vi "HDI Accuracy.vi"() -> ()   [LabVIEW 2011]
uses:
  Shared Components/Gantry Class/Type Definitions/Virtual Modes.ctl
  Shared Components/Gantry Class/Type Definitions/Init_Modes.ctl
  Shared Components/Gantry Class/Gantry Class.lvclass
  Shared Components/Config Manager Class/Type Definitions/Camera Enum.ctl
  Shared Components/Vec3d Class/Vec3d Class.lvclass
panel:
  out "Point being recorded":string="\\P"
  in  "Results Folder":path=path "C:/Users/Admin/Gantry Purdue/pixel-gantry-control/Results"
  out "Iteration Number":i32
  in  "Virtual Mode":T1=enum."Virtual"
  in  "stop":bool
  out "Image":T2(plugin-control)
  out "error out":errorcluster
  in  "Config Folder":path=path "C:/Users/Admin/Gantry Purdue/pixel-gantry-control/Config"
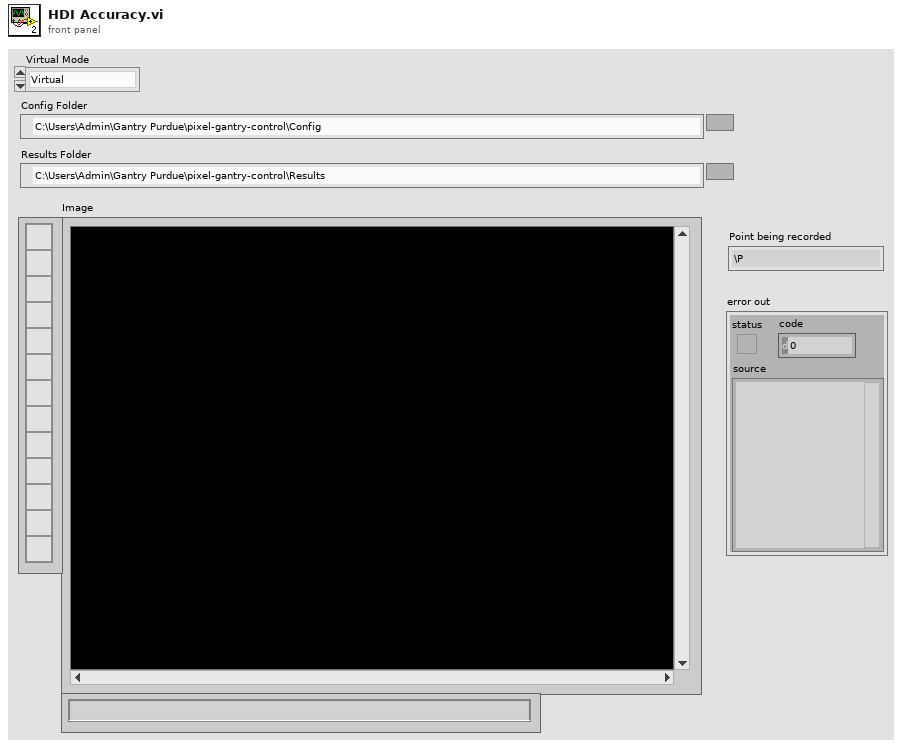
[diagram p1: front panel]
types:
  T1 = typedef "Virtual Modes.ctl" = enum16{"Nonvirtual", "Pseudovirtual", "Virtual"}
  T2 = typedef "IMAQ Image.ctl" = refnum<image>
  T3 = typedef "Init_Modes.ctl" = enum16{"Full", "Robot Only", "Dispenser Only", "Cameras Only", "Robot and Cameras", "Robot and Cameras and Dispenser", "Manifold Only"}
  T4 = typedef "Camera Enum.ctl" = enum16{"GANTRY HEAD", "NEEDLE CALIBRATION X", "NEEDLE CALIBRATION Y", "STAND CAMERA", "SIMRAN WEBCAM"}
  T5 = typedef "Physical Image.ctl" = cluster{"Image Position":refnum<class "Vec3d Class.lvclass">, "Image Reference":T2, "Field of View":cluster{"x(mm)":dbl, "y(mm)":dbl}}
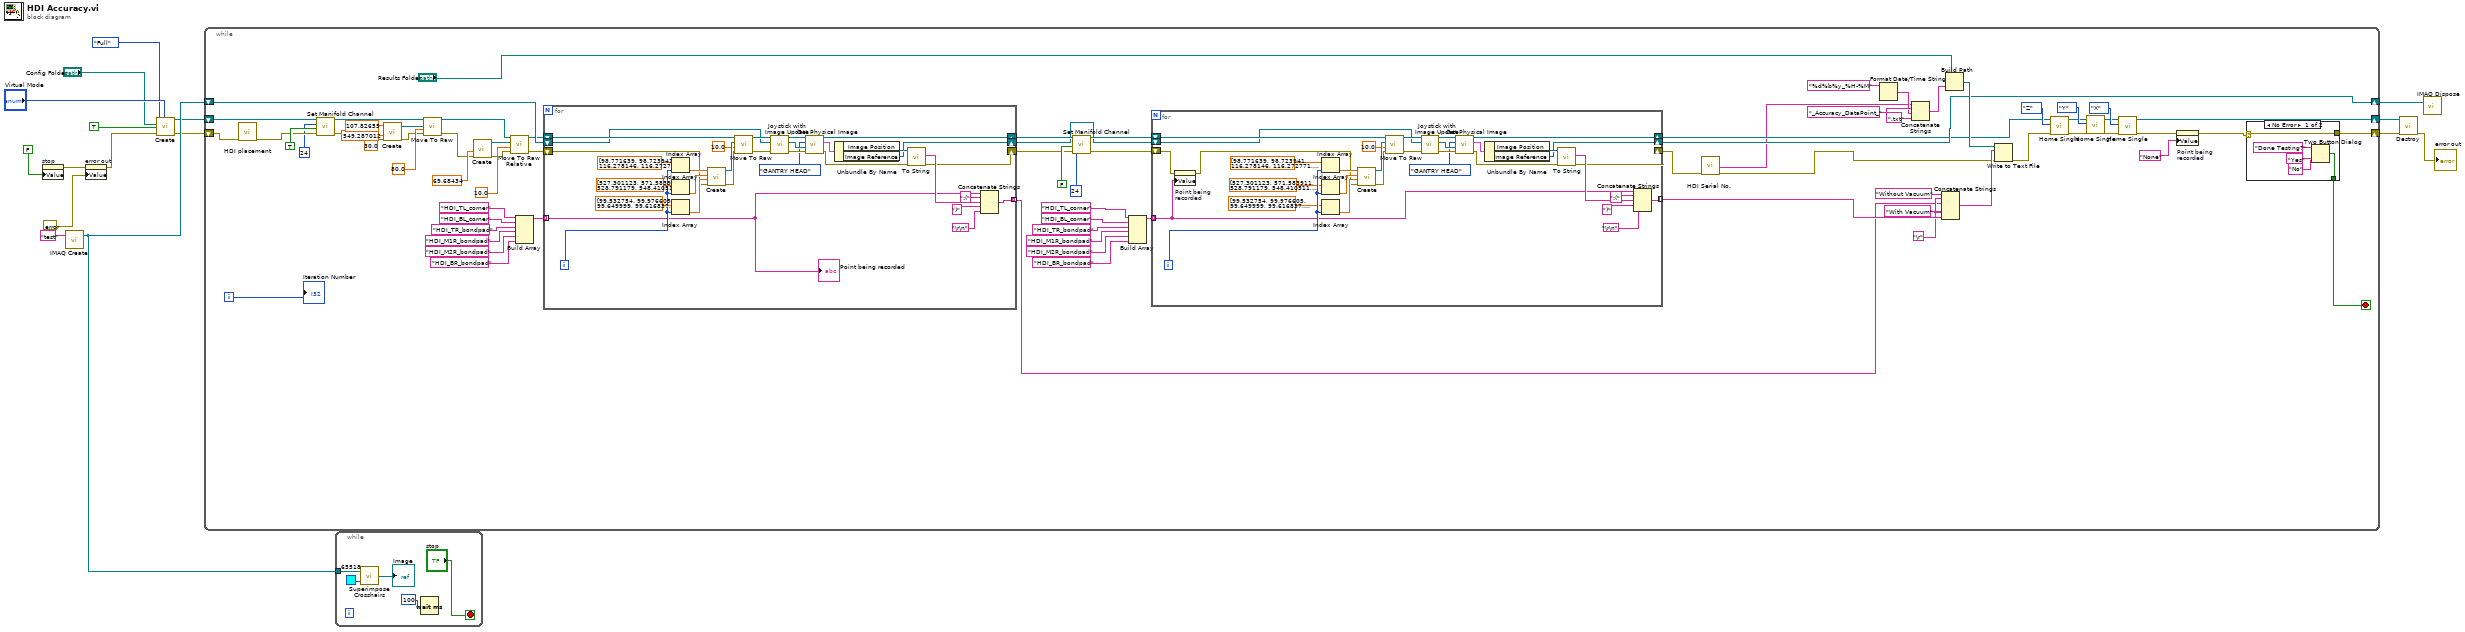
[diagram p0: block diagram]
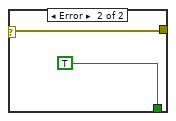
[diagram p2: hidden frame]
diagram:
  n1 = property on="stop" class="Bool (strict)"("Value"=FALSE) -> (error out=w14:errorcluster)  [unwired: 2 in, 1 out]
  n2 = call "IMAQ Create"("Image Name"="test") -> ("New Image"=w11:T2)  [unwired: 4 in, 1 out]
  n3 = property on="error out" class="Clust (strict)"(error in=w14, "Value"=errorcluster {"status"=FALSE, "code"=0, "source"=""} ("error in (no error)")) -> (error out=w9:errorcluster)  [unwired: 1 in, 1 out]
  n4 = call "Create.vi"("Virtual Mode"="Virtual Mode", "error in"=w9, "HOME?"=TRUE, "Config Folder"="Config Folder", "Init Mode"=Init_Modes."Full") -> ("error out"=w6:errorcluster, "Gantry out"=w5:refnum<class "Gantry Class.lvclass">)  [unwired: 5 in]
  n5 = while {
    shift-right: [w34] -> w3
    shift-left: w11 -> [w49]
    shift-right: [w71] -> w2
    shift-left: w5 -> [w76]
    shift-right: [w70] -> w1
    shift-left: w6 -> [w57]
    i -> [w78]
    stop <- w79 stop-if-true
    w37 = "\r"
    n6 = call "HDI placement"("error in (no error)"=w57) -> ("error out"=w74:errorcluster)  [unwired: 17 in, 1 out]
    n7 = call-dynamic "Set Manifold Channel.vi"("error in"=w74, "On/Off"=TRUE, "Manifold Channel"=24, "Gantry in"=w76) -> ("error out"=w73:errorcluster, "Gantry out"=w75:refnum<class "Gantry Class.lvclass">)  [unwired: 6 in]
    n8 = call "Create.vi"("error in"=w73, "Z"=30.0, "Y"=549.287012, "X"=107.82655) -> ("error out"=w89:errorcluster, "Vec3d Class out"=w91:refnum<class "Vec3d Class.lvclass">)  [unwired: 6 in]
    n9 = call-dynamic "Move To Raw.vi"("error in"=w89, "Speed"=80.0, "Destination"=w91, "Gantry in"=w75) -> ("error out"=w47:errorcluster, "Gantry out"=w50:refnum<class "Gantry Class.lvclass">)  [unwired: 6 in]
    n10 = call "Create.vi"("error in"=w47, "Z"=69.68434) -> ("error out"=w58:errorcluster, "Vec3d Class out"=w61:refnum<class "Vec3d Class.lvclass">)  [unwired: 8 in]
    n11 = call-dynamic "Move To Raw Relative.vi"("error in"=w58, "Speed(mm/s)"=10.0, "Delta"=w61, "Gantry in"=w50) -> ("error out"=w48:errorcluster, "Gantry out"=w27:refnum<class "Gantry Class.lvclass">)  [unwired: 6 in]
    n12 = Build Array("HDI_TL_corner" ("string"), "HDI_BL_corner" ("string"), "HDI_TR_bondpad" ("string"), "HDI_M1R_bondpad" ("string"), "HDI_M2R_bondpad" ("string"), "HDI_BR_bondpad" ("string")) -> (w63:string[])
    n13 = for {
      tunnel: [w155] -> w35 mode=indexing
      shift-right: [w156] -> w24
      shift-left: w48 -> [w133]
      shift-right: [w154] -> w22
      shift-left: w27 -> [w149]
      shift-right: [w150] -> w17
      shift-left: w49 -> [w138]
      tunnel: w63 -> [w132] mode=indexing
      i -> [w134]
      n14 = Index Array(array=dbl[] [98.771639, 98.723941, 116.278146, 116.272771, 116.262135, 116.231002, 0.0, 0.0], index=w134) -> (element=w146:dbl)
      n15 = Index Array(array=dbl[] [527.301123, 571.583911, 528.791179, 548.410511, 550.612629, 570.266275, 0.0, 0.0], index=w134) -> (element=w145:dbl)
      n16 = Index Array(array=dbl[] [99.532754, 99.976605, 99.649999, 99.616837, 99.684329, 99.659099, 0.0, 0.0], index=w134) -> (element=w136:dbl)
      n17 = call "Create.vi"("error in"=w133, "Z"=w136, "Y"=w145, "X"=w146) -> ("error out"=w143:errorcluster, "Vec3d Class out"=w144:refnum<class "Vec3d Class.lvclass">)  [unwired: 6 in]
      n18 = call-dynamic "Move To Raw.vi"("error in"=w143, "Speed"=10.0, "Destination"=w144, "Gantry in"=w149) -> ("error out"=w148:errorcluster, "Gantry out"=w147:refnum<class "Gantry Class.lvclass">)  [unwired: 6 in]
      n19 = call-dynamic "Joystick with Image Update.vi"("error in (no error)"=w148, "Image In"=w138, "Gantry Class in"=w147) -> ("error out"=w162:errorcluster, "Image Out"=w153:T2, "Gantry Class out"=w161:refnum<class "Gantry Class.lvclass">)  [unwired: 6 in]
      n20 = call-dynamic "Get Physical Image.vi"("error in"=w162, "Image In"=w153, "Camera Name"=Camera_Enum."GANTRY HEAD", "Gantry in"=w161) -> ("error out"=w135:errorcluster, "Physical Image"=w160:T5, "Gantry out"=w154:refnum<class "Gantry Class.lvclass">)  [unwired: 5 in]
      n21 = Unbundle By Name(w160) -> ("Image Position"=w159:refnum<class "Vec3d Class.lvclass">, "Image Reference"=w150:T2)
      n22 = call "To String.vi"("error in"=w135, "Vec3d in"=w159) -> ("error out"=w156:errorcluster, "Vec3d String"=w157:string)  [unwired: 7 in, 1 out]
      n23 = Concatenate Strings(w132, ":(" ("string"), w157, ")" ("string"), "\r\n" ("string")) -> (w155:string)
      "Point being recorded" <- w132
    }
    n24 = call-dynamic "Set Manifold Channel.vi"("error in"=w24, "On/Off"=FALSE, "Manifold Channel"=24, "Gantry in"=w22) -> ("error out"=w23:errorcluster, "Gantry out"=w21:refnum<class "Gantry Class.lvclass">)  [unwired: 6 in]
    n25 = Build Array("HDI_TL_corner" ("string"), "HDI_BL_corner" ("string"), "HDI_TR_bondpad" ("string"), "HDI_M1R_bondpad" ("string"), "HDI_M2R_bondpad" ("string"), "HDI_BR_bondpad" ("string")) -> (w46:string[])
    n26 = for {
      tunnel: [w124] -> w38 mode=indexing
      shift-right: [w125] -> w30
      shift-left: w23 -> [w105]
      shift-right: [w123] -> w33
      shift-left: w21 -> [w118]
      shift-right: [w119] -> w34
      shift-left: w17 -> [w109]
      tunnel: w46 -> [w104] mode=indexing
      i -> [w106]
      n27 = property on="Point being \nrecorded" class="Str"(error in=w105, "Value"=w104) -> (error out=w103:errorcluster)  [unwired: 1 in, 1 out]
      n28 = Index Array(array=dbl[] [98.771639, 98.723941, 116.278146, 116.272771, 116.262135, 116.231002, 0.0, 0.0], index=w106) -> (element=w115:dbl)
      n29 = Index Array(array=dbl[] [527.301123, 571.583911, 528.791179, 548.410511, 550.612629, 570.266275, 0.0, 0.0], index=w106) -> (element=w114:dbl)
      n30 = Index Array(array=dbl[] [99.532754, 99.976605, 99.649999, 99.616837, 99.684329, 99.659099, 0.0, 0.0], index=w106) -> (element=w108:dbl)
      n31 = call "Create.vi"("error in"=w103, "Z"=w108, "Y"=w114, "X"=w115) -> ("error out"=w112:errorcluster, "Vec3d Class out"=w113:refnum<class "Vec3d Class.lvclass">)  [unwired: 6 in]
      n32 = call-dynamic "Move To Raw.vi"("error in"=w112, "Speed"=10.0, "Destination"=w113, "Gantry in"=w118) -> ("error out"=w117:errorcluster, "Gantry out"=w116:refnum<class "Gantry Class.lvclass">)  [unwired: 6 in]
      n33 = call-dynamic "Joystick with Image Update.vi"("error in (no error)"=w117, "Image In"=w109, "Gantry Class in"=w116) -> ("error out"=w131:errorcluster, "Image Out"=w122:T2, "Gantry Class out"=w130:refnum<class "Gantry Class.lvclass">)  [unwired: 6 in]
      n34 = call-dynamic "Get Physical Image.vi"("error in"=w131, "Image In"=w122, "Camera Name"=Camera_Enum."GANTRY HEAD", "Gantry in"=w130) -> ("error out"=w107:errorcluster, "Physical Image"=w129:T5, "Gantry out"=w123:refnum<class "Gantry Class.lvclass">)  [unwired: 5 in]
      n35 = Unbundle By Name(w129) -> ("Image Position"=w128:refnum<class "Vec3d Class.lvclass">, "Image Reference"=w119:T2)
      n36 = call "To String.vi"("error in"=w107, "Vec3d in"=w128) -> ("error out"=w125:errorcluster, "Vec3d String"=w126:string)  [unwired: 7 in, 1 out]
      n37 = Concatenate Strings(w104, ":(" ("string"), w126, ")" ("string"), "\r\n" ("string")) -> (w124:string)
    }
    n38 = call "HDI Serial No."("error in (no error)"=w30) -> ("Serial No."=w28:string, "error out"=w29:errorcluster)  [unwired: 16 in, 1 out]
    n39 = Format Date/Time String(time format string (%c)="%d%b%y_%H-%M") -> (date/time string=w64:string)  [unwired: 2 in]
    n40 = Concatenate Strings(w28, "_Accuracy_DataPoint_" ("name or relative path"), w64, ".txt" ("string")) -> (w66:string)
    n41 = Concatenate Strings("Without Vacuum" ("string"), w37, w35, "With Vacuum" ("string"), w37, w38) -> (w62:string)
    n42 = Build Path(base path="Results Folder", name or relative path=w66) -> (appended path=w69:path)
    n43 = Write to Text File(file (use dialog)=w69, text=w62, error in=w29) -> (error out=w32:errorcluster)  [unwired: 1 in, 2 out]
    n44 = call-dynamic "Home Single.vi"("error in"=w32, "Axis"=enum16{"X", "Y", "Z", "U"}."Z", "Gantry in"=w33) -> ("error out"=w84:errorcluster, "Gantry out"=w85:refnum<class "Gantry Class.lvclass">)  [unwired: 7 in]
    n45 = call-dynamic "Home Single.vi"("error in"=w84, "Axis"=enum16{"X", "Y", "Z", "U"}."Y", "Gantry in"=w85) -> ("error out"=w82:errorcluster, "Gantry out"=w83:refnum<class "Gantry Class.lvclass">)  [unwired: 7 in]
    n46 = call-dynamic "Home Single.vi"("error in"=w82, "Axis"=enum16{"X", "Y", "Z", "U"}."X", "Gantry in"=w83) -> ("error out"=w20:errorcluster, "Gantry out"=w71:refnum<class "Gantry Class.lvclass">)  [unwired: 7 in]
    n47 = property on="Point being\nrecorded" class="Str"(error in=w20, "Value"="None" ("Point being recorded")) -> (error out=w19:errorcluster)  [unwired: 1 in, 1 out]
    n48 = case shown="No Error" w19 {
      selector: w19 -> [w93 w99]
      tunnel: [w93 w99] -> w70
      tunnel: [w94 TRUE ("Done Testing?")] -> w79
      frame No Error {
        n49 = Two Button Dialog(message="Done Testing?", 1:"No" ("F button name (\"Cancel\")"), 2:"Yes" ("T button name (\"OK\")")) -> (T button?=w94:bool)
      }
      frame Error {
      }
    }
    "Iteration Number" <- w78
  }
  n50 = while {
    tunnel: w11 -> [w165]
    stop <- "stop" stop-if-true
    n51 = call "Superimpose Crosshairs.vi"("Grid Line Color"=u32 65518, "Refnum in"=w165) -> ("Refnum out"=→"Image":T2)
    n52 = Wait (ms)(milliseconds to wait=u32 100) -> ()  [unwired: 1 out]
  }
  n53 = call "Destroy.vi"("error in"=w1, "Gantry Class in"=w2) -> ("error out"=→"error out":errorcluster)  [unwired: 9 in]
  n54 = call "IMAQ Dispose"("Image"=w3) -> ()  [unwired: 5 in, 1 out]
